vi "Validate.vi"(6 "Length":u8, 8 "error in":errorcluster, 9 "Sub-Index":i16 format="%.0x", 10 "Index":u16 format="%.0x", 11 "EDS":refnum<class "Electronic Datasheet.lvclass">) -> (0 "error out":errorcluster, 1 "Valid?":bool, 2 "Mapping Target":refnum<class "OD Entry.lvclass">)   [LabVIEW 2019, in "PDO Grid.lvlib" / "PDO Mapping.lvclass"]
uses:
  PDO Mapping.lvclass
  Electronic Datasheet/Electronic Datasheet.lvclass
  Core/OD Entry/OD Entry.lvclass
  PDO Grid.lvlib
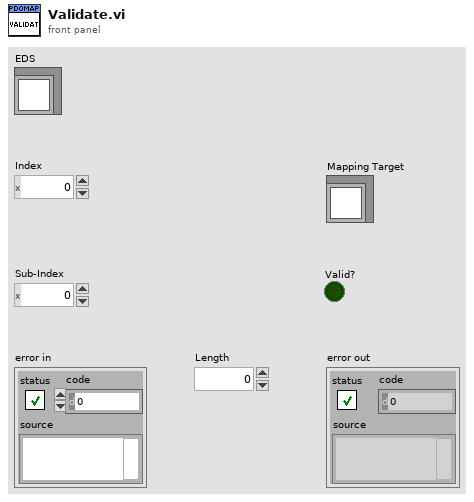
[diagram p1: front panel]
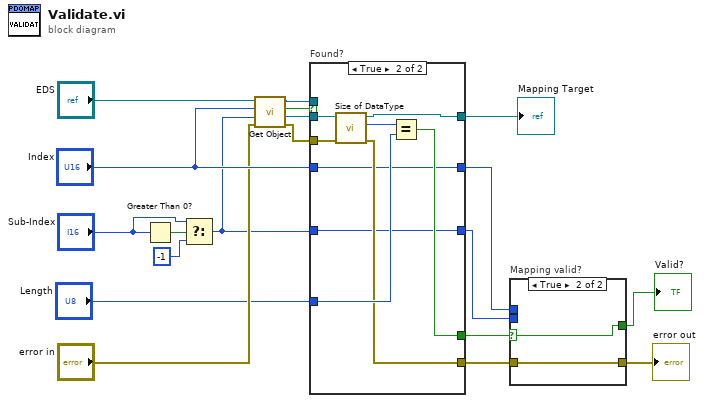
[diagram p0: block diagram]
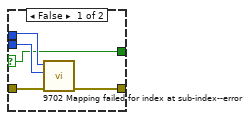
[diagram p3: hidden frame]
diagram:
  n1 = Greater Than 0?(x="Sub-Index") -> (x > 0?=w16:bool)
  n2 = Select(t="Sub-Index", s=w16, f=i16 -1) -> (s? t:f=w12:i16)
  n3 = call "Get Object.vi"("error in"="error in", "Sub-Index"=w12, "Index"="Index", "reference in"="EDS") -> ("error out"=w8:errorcluster, "OD Entry"=w9:refnum<class "OD Entry.lvclass">, "Found?"=w17:bool, "reference out"=w10:refnum<class "Electronic Datasheet.lvclass">)  [unwired: 4 in]
  n4 = case "Found?" shown="True" w17 {
    selector: w17 -> [w20 _]
    tunnel: [w21 w27] -> w7
    tunnel: "Index" -> [w23 w26]
    tunnel: w12 -> [w22 w25]
    tunnel: "Length" -> [_ w29]
    tunnel: w10 -> [_ _]
    tunnel: w9 -> [_ w32]
    tunnel: w8 -> [w21 w31]
    tunnel: [w20 w28] -> w5
    tunnel: [w23 w26] -> w4
    tunnel: [w22 w25] -> w3
    tunnel: [_ w24] -> w1
    frame False {
    }
    frame True {
      n5 = call "Size of DataType.vi"("error in"=w31, "OD Entry in"=w32) -> ("error out"=w27:errorcluster, "Size in Bits"=w30:i32, "OD Entry out"=w24:refnum<class "OD Entry.lvclass">)  [unwired: 7 in]
      n6 = Equal?(x=w30, y=w29) -> (x = y?=w28:bool)
    }
  }
  "Mapping Target" <- w1
  n7 = case "Mapping valid?" shown="True" w5 {
    selector: w5 -> [w33 w38]
    tunnel: w7 -> [w37 w39]
    tunnel: [w36 w39] -> w6
    tunnel: w4 -> [w35 _]
    tunnel: w3 -> [w34 _]
    tunnel: [w33 w38] -> w2
    frame False {
      n8 = call "9702 Mapping failed for index at sub-index--error.vi"("error in (no error)"=w37, "Sub-Index"=w34, "Index"=w35) -> ("error out"=w36:errorcluster)  [unwired: 8 in]
    }
    frame True {
    }
  }
  "error out" <- w6
  "Valid?" <- w2
